vi "Setscan_advanced_output.vi"(8 "error in (no error)":errorcluster, 10 "Set_Val":T1, 11 "OneOfTemplate in":refnum<class "niswitch_grpc_ConfigureScanTriggerRequest_scan_advanced_output_enum.lvclass">) -> (0 "error out":errorcluster, 3 "OneOfTemplate out":refnum<class "niswitch_grpc_ConfigureScanTriggerRequest_scan_advanced_output_enum.lvclass">)   [LabVIEW 2021, in "NI Switch_client.lvlib" / "niswitch_grpc_ConfigureScanTriggerRequest_scan_advanced_output_enum.lvclass"]
uses:
  niswitch_grpc_ConfigureScanTriggerRequest_scan_advanced_output_enum.lvclass
  niswitch_grpc_ScanAdvancedOutput.ctl
  niswitch_grpc_ConfigureScanTriggerRequest_scan_advanced_output_enum.lvclass/niswitch_grpc_ConfigureScanTriggerRequest_scan_advanced_output_enum.ctl
  NI Switch_client.lvlib
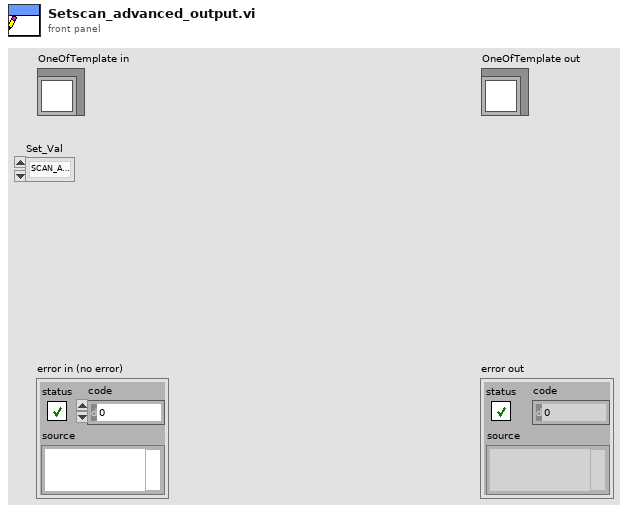
[diagram p1: front panel]
types:
  T1 = typedef "NI Switch_client.lvlib/niswitch_grpc_ScanAdvancedOutput.ctl" = enum32{"SCAN_ADVANCED_OUTPUT_NISWITCH_VAL_NONE", "SCAN_ADVANCED_OUTPUT_NISWITCH_VAL_EXTERNAL", "SCAN_ADVANCED_OUTPUT_NISWITCH_VAL_TTL0", "SCAN_ADVANCED_OUTPUT_NISWITCH_VAL_TTL1", "SCAN_ADVANCED_OUTPUT_NISWITCH_VAL_TTL2", "SCAN_ADVANCED_OUTPUT_NISWITCH_VAL_TTL3", "SCAN_ADVANCED_OUTPUT_NISWITCH_VAL_TTL4", "SCAN_ADVANCED_OUTPUT_NISWITCH_VAL_TTL5", "SCAN_ADVANCED_OUTPUT_NISWITCH_VAL_TTL6", "SCAN_ADVANCED_OUTPUT_NISWITCH_VAL_TTL7", "SCAN_ADVANCED_OUTPUT_NISWITCH_VAL_PXI_STAR", "SCAN_ADVANCED_OUTPUT_NISWITCH_VAL_REARCONNECTOR", "SCAN_ADVANCED_OUTPUT_NISWITCH_VAL_FRONTCONNECTOR", "SCAN_ADVANCED_OUTPUT_NISWITCH_VAL_REARCONNECTOR_MODULE1", "SCAN_ADVANCED_OUTPUT_NISWITCH_VAL_REARCONNECTOR_MODULE2", "SCAN_ADVANCED_OUTPUT_NISWITCH_VAL_REARCONNECTOR_MODULE3", "SCAN_ADVANCED_OUTPUT_NISWITCH_VAL_REARCONNECTOR_MODULE4", "SCAN_ADVANCED_OUTPUT_NISWITCH_VAL_REARCONNECTOR_MODULE5", "SCAN_ADVANCED_OUTPUT_NISWITCH_VAL_REARCONNECTOR_MODULE6", "SCAN_ADVANCED_OUTPUT_NISWITCH_VAL_REARCONNECTOR_MODULE7", "SCAN_ADVANCED_OUTPUT_NISWITCH_VAL_REARCONNECTOR_MODULE8", "SCAN_ADVANCED_OUTPUT_NISWITCH_VAL_REARCONNECTOR_MODULE9", "SCAN_ADVANCED_OUTPUT_NISWITCH_VAL_REARCONNECTOR_MODULE10", "SCAN_ADVANCED_OUTPUT_NISWITCH_VAL_REARCONNECTOR_MODULE11", "SCAN_ADVANCED_OUTPUT_NISWITCH_VAL_REARCONNECTOR_MODULE12", "SCAN_ADVANCED_OUTPUT_NISWITCH_VAL_FRONTCONNECTOR_MODULE1", "SCAN_ADVANCED_OUTPUT_NISWITCH_VAL_FRONTCONNECTOR_MODULE2", "SCAN_ADVANCED_OUTPUT_NISWITCH_VAL_FRONTCONNECTOR_MODULE3", "SCAN_ADVANCED_OUTPUT_NISWITCH_VAL_FRONTCONNECTOR_MODULE4", "SCAN_ADVANCED_OUTPUT_NISWITCH_VAL_FRONTCONNECTOR_MODULE5", "SCAN_ADVANCED_OUTPUT_NISWITCH_VAL_FRONTCONNECTOR_MODULE6", "SCAN_ADVANCED_OUTPUT_NISWITCH_VAL_FRONTCONNECTOR_MODULE7", "SCAN_ADVANCED_OUTPUT_NISWITCH_VAL_FRONTCONNECTOR_MODULE8", "SCAN_ADVANCED_OUTPUT_NISWITCH_VAL_FRONTCONNECTOR_MODULE9", "SCAN_ADVANCED_OUTPUT_NISWITCH_VAL_FRONTCONNECTOR_MODULE10", "SCAN_ADVANCED_OUTPUT_NISWITCH_VAL_FRONTCONNECTOR_MODULE11", "SCAN_ADVANCED_OUTPUT_NISWITCH_VAL_FRONTCONNECTOR_MODULE12"}
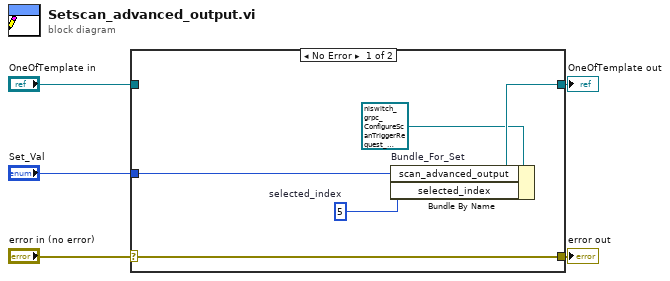
[diagram p0: block diagram]
diagram:
  n1 = case shown="No Error" "error in (no error)" {
    selector: "error in (no error)" -> [w10 w11]
    tunnel: [w10 w11] -> w4
    tunnel: [w9 w12] -> w2
    tunnel: "OneOfTemplate in" -> [_ w12]
    tunnel: "Set_Val" -> [w8 _]
    frame No Error {
      w7 = 5  # selected_index
      n2 = Bundle By Name "Bundle_For_Set"(cluster=refnum<class "niswitch_grpc_ConfigureScanTriggerRequest_scan_advanced_output_enum.lvclass"> refnum ("OneOfTemplate in"), "scan_advanced_output"=w8, "selected_index"=w7) -> (w9:refnum<class "niswitch_grpc_ConfigureScanTriggerRequest_scan_advanced_output_enum.lvclass">)
    }
    frame Error {
    }
  }
  "error out" <- w4
  "OneOfTemplate out" <- w2
